vi "runTest.vi"(8 "error in (no error)":errorcluster, 11 "TestCase in":refnum<class "MyFirstTest.lvclass">) -> (0 "error out":errorcluster, 3 "TestCase out":refnum<class "MyFirstTest.lvclass">)   [LabVIEW 2011, in "MyFirstTest.lvclass"]
uses:
  MyFirstTest.lvclass
panel:
  # "Copyright © 2007 James Kring, Inc. All rights reserved.\n\nAuthor: Jim Kring [jim.kring@jameskring.com]\n\nThis library is provided \"AS IS\" ,WITHOUT WARRANTIES OR \nCONDITIONS OF ANY KIND, either express or implied.\n\nJames Kring, Inc. -- http://www.jameskring.com"
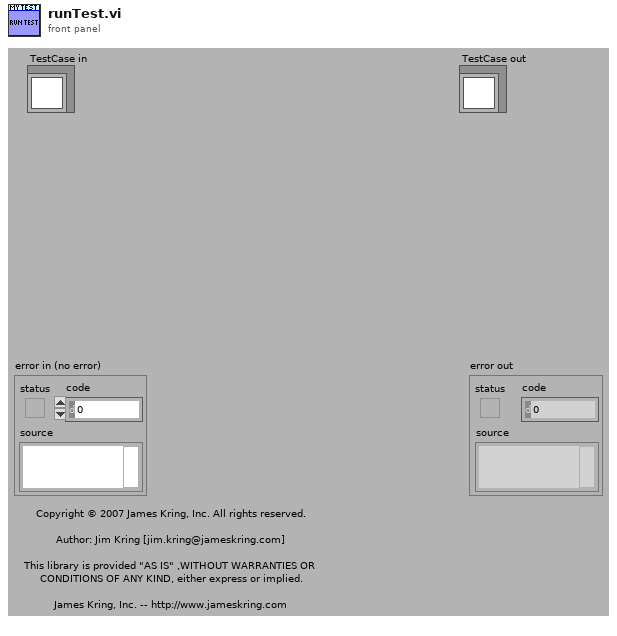
[diagram p1: front panel]
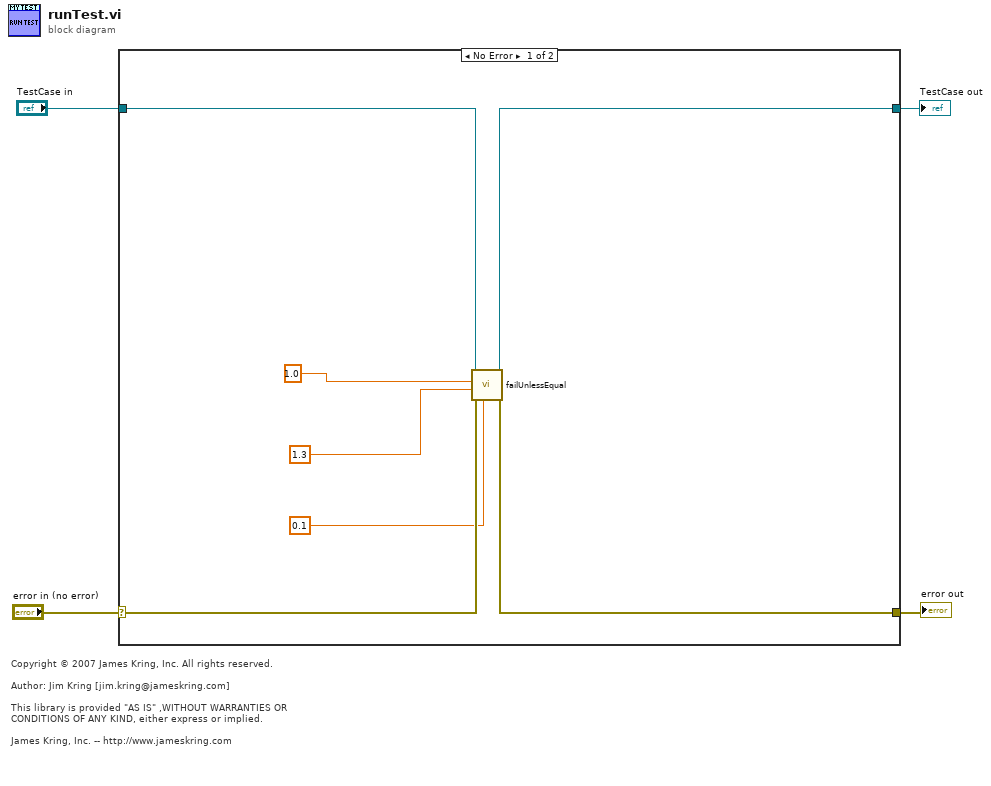
[diagram p0: block diagram]
diagram:
  # "Copyright © 2007 James Kring, Inc. All rights reserved.\n\nAuthor: Jim Kring [jim.kring@jameskring.com]\n\nThis library is provided \"AS IS\" ,WITHOUT WARRANTIES OR \nCONDITIONS OF ANY KIND, either express or implied.\n\nJames Kring, Inc. -- http://www.jameskring.com"
  n1 = case shown="No Error" "error in (no error)" {
    selector: "error in (no error)" -> [w11 w13]
    tunnel: [w10 w13] -> w3
    tunnel: [w6 w12] -> w1
    tunnel: "TestCase in" -> [w5 w12]
    frame No Error {
      n2 = call-dynamic "failUnlessEqual.vi"("delta (optional)"=0.1, "error in (no error)"=w11, "y"=1.3, "x"=1.0, "TestCase in"=w5) -> ("error out"=w10:errorcluster, "TestCase out"=w6:refnum<class "MyFirstTest.lvclass">)  [unwired: 5 in]
    }
    frame Error {
    }
  }
  "error out" <- w3
  "TestCase out" <- w1
